vi "Update Configuration.vi"(8 "error in (no error)":errorcluster, 11 "CIFTemplateNode in":refnum<class "CIFCorePlugin.lvclass">) -> (0 "error out":errorcluster, 3 "CIFTemplateNode out":refnum<class "CIFCorePlugin.lvclass">)   [LabVIEW 2021, in "CIFCorePlugin.lvclass"]
uses:
  CIFCorePlugin.lvclass
  CIFCorePlugin.lvclass/CIFCorePlugin.ctl
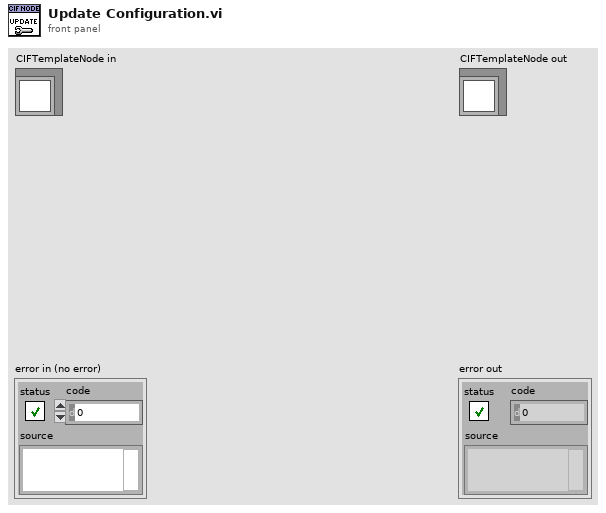
[diagram p1: front panel]
types:
  T1 = typedef "CIFCoreCommon.lvlib/Common Plugin Configuration.ctl" = cluster{"Period (s)":dbl, "Offset (us)":i32, "Priority":i32, "Processor":i32, "External Clock":T2}
  T2 = typedef "CIFCoreCommon.lvlib/External Clock Config.ctl" = cluster{"ClockID":u8, "Clock Name":string, "Publish Clock":bool, "Convert Data Timestamps":bool, "Plugin Timing Source":bool}
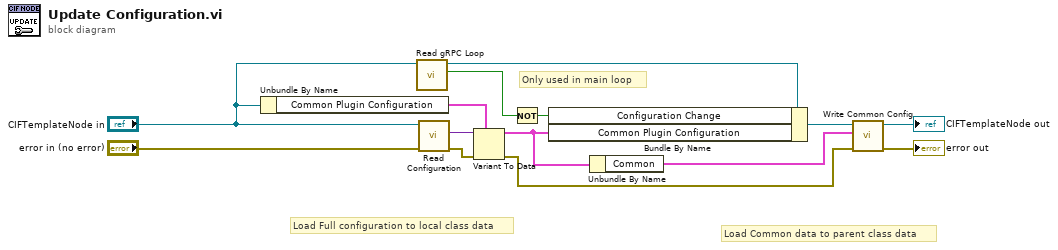
[diagram p0: block diagram]
diagram:
  # "Only used in main loop"
  # "Load Common data to parent class data"
  # "Load Full configuration to local class data"
  n1 = Unbundle By Name("CIFTemplateNode in") -> ("Common Plugin Configuration"=w8:cluster{"Common":T1})
  n2 = call "Read gRPC Loop.vi"("CIFCorePlugin in"="CIFTemplateNode in") -> ("gRPC Loop"=w2:bool, "CIFCorePlugin out"=w3:refnum<class "CIFCorePlugin.lvclass">)  [unwired: 8 in, 1 out]
  n3 = call "Read Configuration.vi"("error in"="error in (no error)", "CIFCorePlugin in"="CIFTemplateNode in") -> ("error out"=w6:errorcluster, "Configuration Data"=w7:variant)  [unwired: 7 in, 1 out]
  n4 = Variant To Data(error in=w6, type=w8, Variant=w7) -> (data=w5:cluster{"Common":T1}, error out=w11:errorcluster)
  n5 = Not(x=w2) -> (.not. x?=w1:bool)
  n6 = Bundle By Name(cluster=w3, "Configuration Change"=w1, "Common Plugin Configuration"=w5) -> (w13:refnum<class "CIFCorePlugin.lvclass">)
  n7 = Unbundle By Name(w5) -> ("Common"=w12:T1)
  n8 = call "Write Common Config.vi"("error in (no error)"=w11, "Common"=w12, "CIFTemplateNode in"=w13) -> ("error out"=→"error out":errorcluster, "CIFTemplateNode out"=→"CIFTemplateNode out":refnum<class "CIFCorePlugin.lvclass">)  [unwired: 7 in]
